vi "Create or Load Experiment Dialog.vi"(8 "error in (no error)":errorcluster, 11 "User Preferences File.lvclass":refnum<class "User Preferences File.lvclass">) -> (0 "error out":errorcluster, 1 "Cancelled?":bool, 2 "Experimental File Cluster":T1, 3 "Experiment File Path":path, 4 "Experiment File Extension":string, 5 "Experiment Name":string)   [LabVIEW 2020, in "RxnRover.lvlib" / "Experiment Manager.lvlib"]
uses:
  Experiment Manager.lvlib
  Experiment File/Experiment File Cluster.ctl
  Plugin Servers/Controller/Minimal Controller Cluster.ctl
  Plugin Servers/Parameter to Hardware Map/Minimal Map.ctl
  Plugin Servers/Parameter to Hardware Map/Minimal Pair Cluster.ctl
  UI Data.ctl
  Sub VIs/Message Queue/Enqueue Message (Single).vi
  <vilib>/Utility/error.llb/Error Cluster From Error Code.vi
  <vilib>/ErrorRing/Error Ring.xnode
  User Preferences/User Preferences File.lvclass
  Sub VIs/Message Queue/test Message Queue.lvlib
  User Event - Stop/User Event - Stop.lvlib
  Plugin Servers/Controller/Generic Plugin.lvclass
  Experiment File/Experiment File.lvlib
  Plugin Servers/Parameter to Hardware Map/Parameter to Hardware Map.lvclass
panel:
  in  "Continue Without Experiment Btn":bool
  in  "Load Experiment Btn":bool
  in  "New Experiment Btn":bool
  in  "Clear Recent Experiments Button":bool
  in  "Recent Experiments Listbox":i32(listbox)
  # "Create or Load Experiment"
  # "Experiment Options"
  # "Recent Experiments"
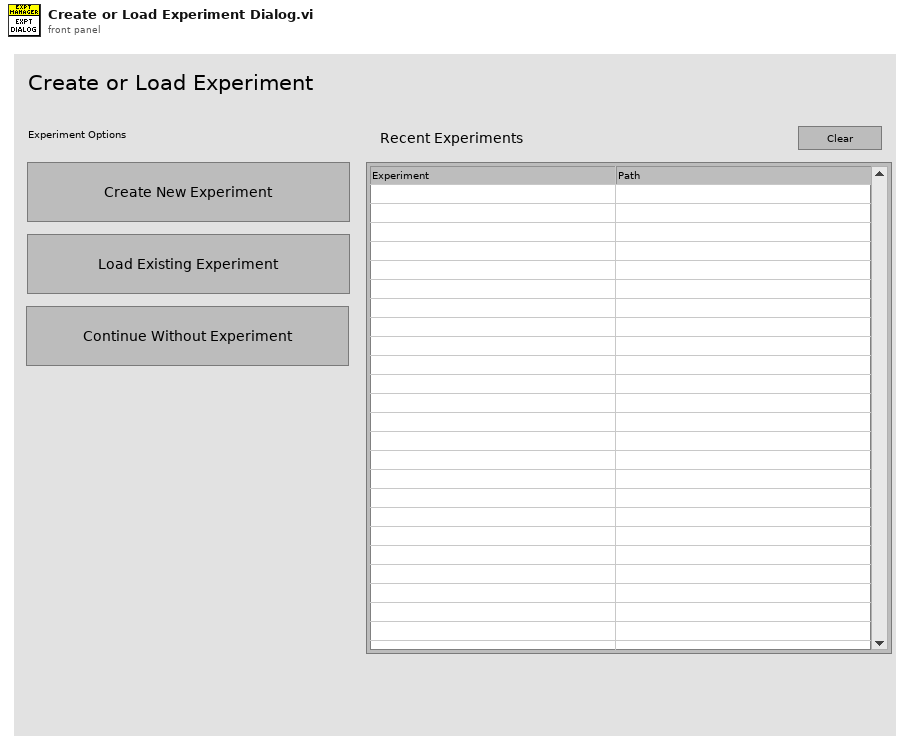
[diagram p1: front panel]
types:
  T1 = typedef "RxnRover.lvlib/Experiment File.lvlib/Experiment File Cluster.ctl" = cluster{"Hardware List":T2[], "Optimizer List":T2[], "Analyzer List":T2[], "Parameter to Hardware Map":T3}
  T2 = typedef "RxnRover.lvlib/Generic Plugin.lvclass/Minimal Controller Cluster.ctl" = cluster{"Name":string, "Controller Type":string, "Control Panel Path":string, "Resource":string}
  T3 = typedef "RxnRover.lvlib/Parameter to Hardware Map.lvclass/Minimal Map.ctl" = T4[]
  T4 = typedef "RxnRover.lvlib/Parameter to Hardware Map.lvclass/Minimal Pair Cluster.ctl" = cluster{"key":string, "values":T2[]}
  T5 = typedef "RxnRover.lvlib/Experiment Manager.lvlib/UI Data.ctl" = cluster{"New Project Btn":refnum<vi>, "Load Project Btn":refnum<vi>, "Cancelled?":bool, "Experiment File Path":path, "Experiment File":T1, "Experiment Directory":path, "Experiment Name":string, "Experiment File Extension":string, "User Preferences File":refnum<class "User Preferences File.lvclass">, "Recent Experiments Listbox":refnum<vi>}
  T6 = enum32{"Invalid", "Standard", "Closed", "Hidden", "Minimized", "Maximized"}
  T7 = typedef "RxnRover.lvlib/User Preferences File.lvclass/User Preferences Cluster.ctl" = cluster{"Max Recent Experiments":dbl, "Recent Experiments":string[], "Log Level":string}
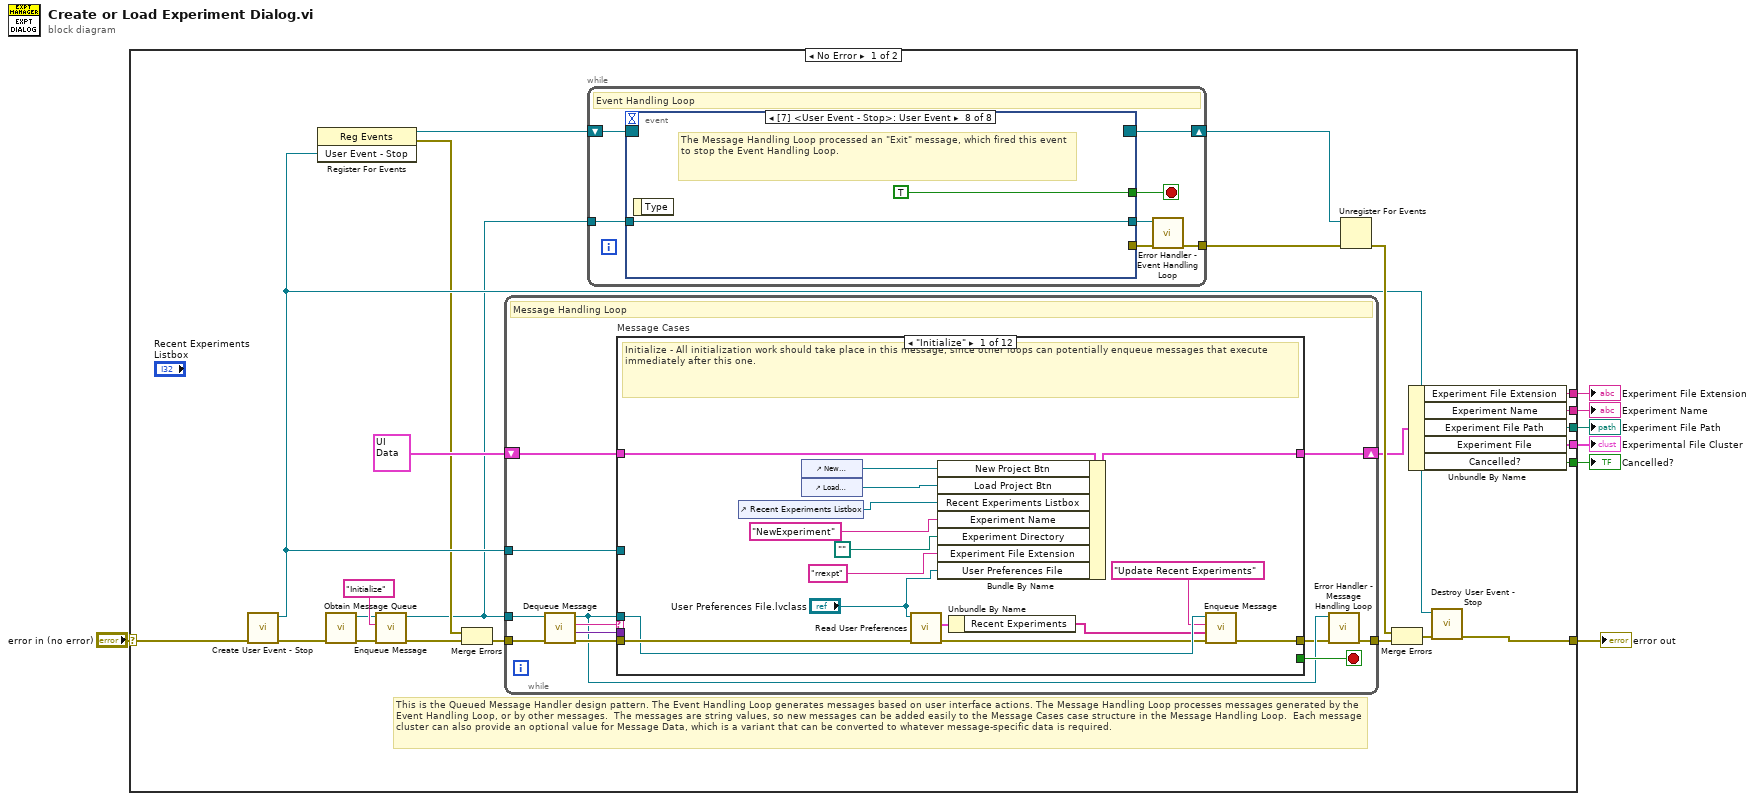
[diagram p0: block diagram]
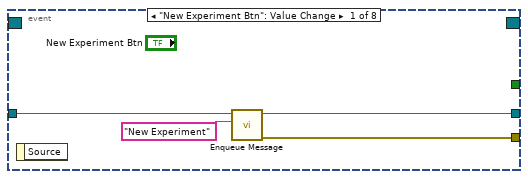
[diagram p2: hidden frame]
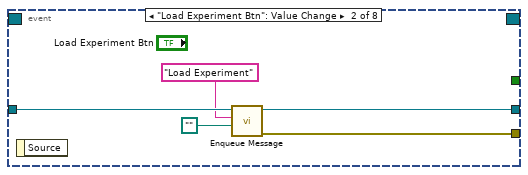
[diagram p3: hidden frame]
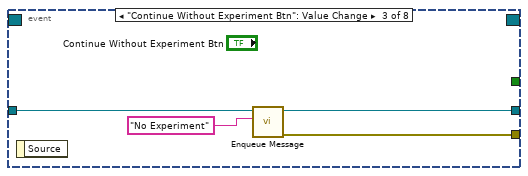
[diagram p4: hidden frame]
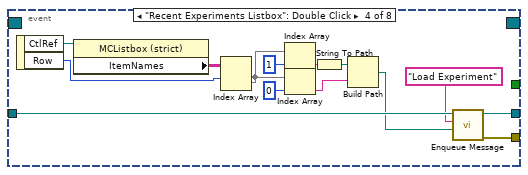
[diagram p5: hidden frame]
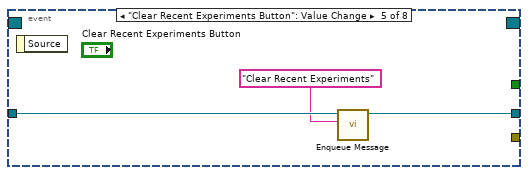
[diagram p6: hidden frame]
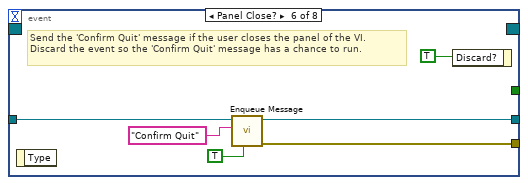
[diagram p7: hidden frame]
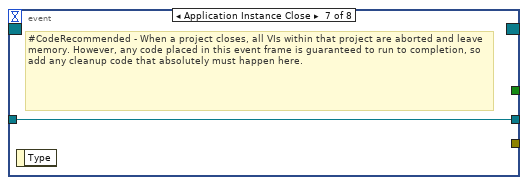
[diagram p8: hidden frame]
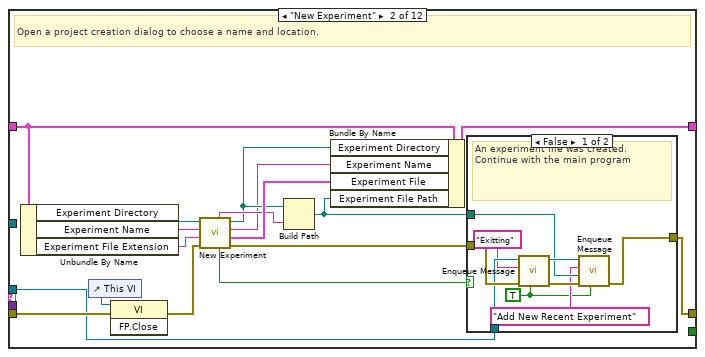
[diagram p9: hidden frame]
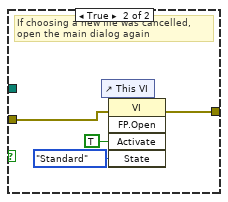
[diagram p10: hidden frame]
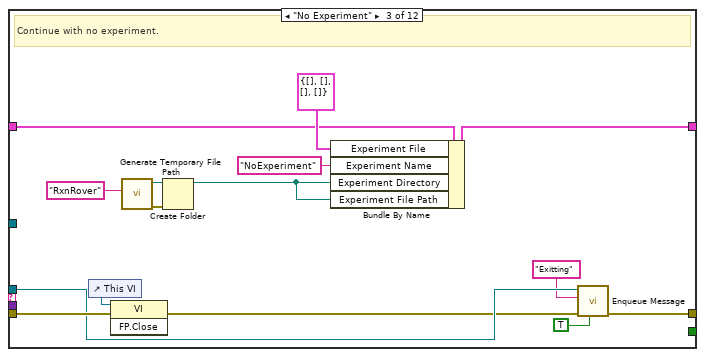
[diagram p11: hidden frame]
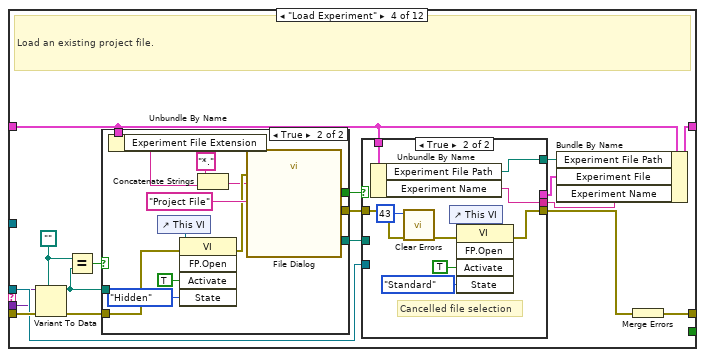
[diagram p12: hidden frame]
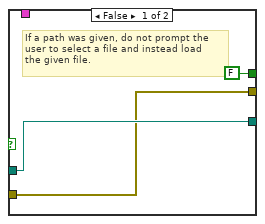
[diagram p13: hidden frame]
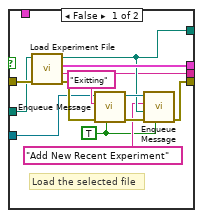
[diagram p14: hidden frame]
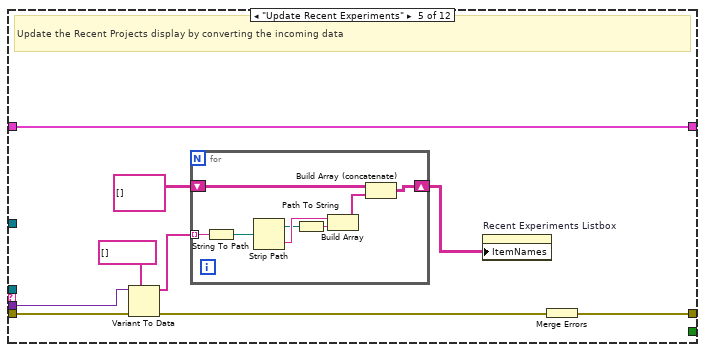
[diagram p15: hidden frame]
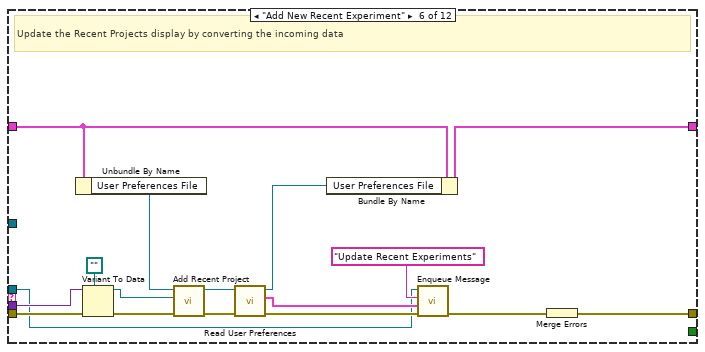
[diagram p16: hidden frame]
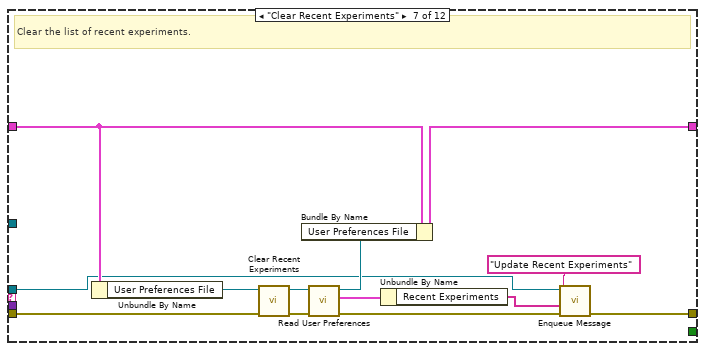
[diagram p17: hidden frame]
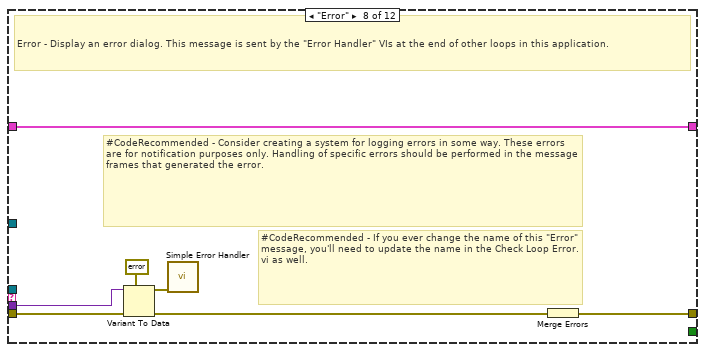
[diagram p18: hidden frame]
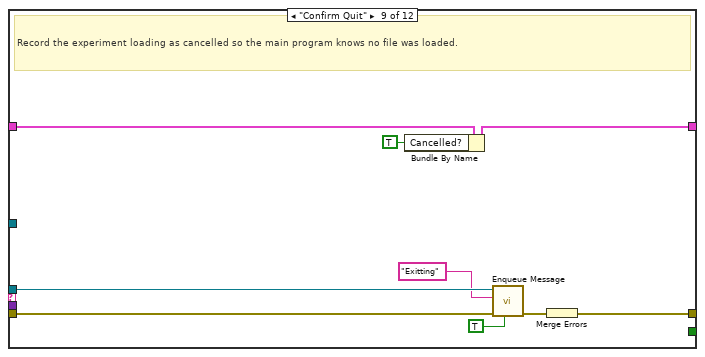
[diagram p19: hidden frame]
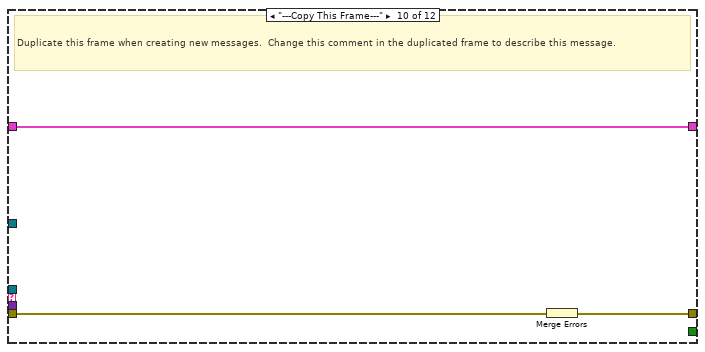
[diagram p20: hidden frame]
diagram:
  n1 = case shown="No Error" "error in (no error)" {
    selector: "error in (no error)" -> [w11 w301]
    tunnel: [w15 w301] -> w1
    tunnel: [w13 T1 {"Hardware List"=[], "Optimizer List"=[], "Analyzer List"=[], "Parameter to Hardware Map"=[]} ("File")] -> w7
    tunnel: [w12 TRUE ("Cancelled?")] -> w6
    tunnel: [w10 path ""] -> w4
    tunnel: [w9 w297] -> w3
    tunnel: [w8 w297] -> w2
    frame No Error {
      # "This is the Queued Message Handler design pattern. The Event Handling Loop generates messages based on user interface actions. The Message Handling Loop processes messages generated by the Event Handling Loop, or by other messages.  The messages are string values, so new messages can be added easily to the Message Cases case structure in the Message Handling Loop.  Each message cluster can also provide an optional value for Message Data, which is a variant that can be converted to whatever message-specific data is required."
      n2 = call "Create User Event - Stop.vi"("error in (no error)"=w11) -> ("error out"=w21:errorcluster, "User Event - Stop"=w24:refnum<user-event>)  [unwired: 9 in]
      n3 = register-events(w24) -> (reference out=w25:refnum<event-registration>, error out=w22:errorcluster)  [unwired: 2 in]
      n4 = call "Obtain Message Queue.vi"("error in (no error)"=w21) -> ("error out"=w20:errorcluster, "Message Queue"=w17:refnum<queue>)  [unwired: 9 in]
      n5 = call-poly "Enqueue Message.vi"("error in (no error)"=w20, "Message"="Initialize", "Message Queue"=w17) -> ("error out"=w19:errorcluster, "dup Message Queue"=w16:refnum<queue>)  [unwired: 7 in]
      n6 = Merge Errors(w22, w19) -> (w23:errorcluster)
      n7 = while {
        tunnel: w16 -> [w81]
        shift-right: [w88] -> w14
        shift-left: T5 {"New Project Btn"=refnum, "Load Project Btn"=refnum, "Cancelled?"=FALSE, "Experiment File Path"=path "", "Experiment File"={"Hardware List"=[], "Optimizer List"=[], "Analyzer List"=[], "Parameter to Hardware Map"=[]}, "Experiment Directory"=path "", "Experiment Name"="", "Experiment File Extension"="", "User Preferences File"=refnum, "Recent Experiments Listbox"=refnum} ("Data Cluster") -> [w89]
        tunnel: w24 -> [w86]
        tunnel: w23 -> [w85]
        tunnel: [w79] -> w31
        stop <- w87 stop-if-true
        # "Message Handling Loop"
        n8 = call "Dequeue Message.vi"("error in (no error)"=w85, "Message Queue"=w81) -> ("error out"=w84:errorcluster, "Message Data"=w82:variant, "Message"=w83:string, "dup Message Queue"=w80:refnum<queue>)  [unwired: 6 in]
        n9 = case "Message Cases" shown="\"Initialize\"" w83 {
          selector: w83 -> [_ _ _ _ _ _ _ _ _ _ _ w287]
          tunnel: w80 -> [w99 w116 w148 w158 _ w226 w244 _ w266 _ w286 _]
          tunnel: w84 -> [w104 w120 w149 w162 w214 w240 w254 w261 w270 w273 w280 _]
          tunnel: [w105 w117 w145 w168 w215 w241 w245 w255 w268 w271 w283 w288] -> w78
          tunnel: w89 -> [w103 w115 w139 w159 w216 w237 w253 w260 w269 w272 w276 w289]
          tunnel: [w102 w122 w151 w163 w216 w232 w251 w260 w263 w272 w276 w289] -> w88
          tunnel: [_ _ _ _ _ _ _ _ _ _ TRUE _] -> w87
          tunnel: w82 -> [_ _ _ w156 w213 w239 _ w259 _ _ w277 _]
          tunnel: w86 -> [_ _ _ _ _ _ _ _ _ _ w282 _]
          frame "Initialize" {
            # "Initialize - All initialization work should take place in this message, since other loops can potentially enqueue messages that execute immediately after this one."
            n10 = control-ref of="Recent Experiments Listbox"() -> (w91:refnum<vi>)
            n11 = control-ref of="New Experiment Btn"() -> (w101:refnum<vi>)
            n12 = control-ref of="Load Experiment Btn"() -> (w100:refnum<vi>)
            n13 = call-dynamic "Read User Preferences.vi"("error in (no error)"=w104, "User Preferences File in"="User Preferences File.lvclass") -> ("error out"=w94:errorcluster, "User Preferences"=w93:T7)  [unwired: 7 in, 1 out]
            n14 = Bundle By Name(cluster=w103, "New Project Btn"=w101, "Load Project Btn"=w100, "Recent Experiments Listbox"=w91, "Experiment Name"="NewExperiment", "Experiment Directory"=path "", "Experiment File Extension"="rrexpt", "User Preferences File"="User Preferences File.lvclass") -> (w102:T5)
            n15 = Unbundle By Name(w93) -> ("Recent Experiments"=w92:string[])
            n16 = call-poly "Enqueue Message.vi"("error in (no error)"=w94, "Message Data"=w92, "Message"="Update Recent Experiments", "Message Queue"=w99) -> ("error out"=w105:errorcluster)  [unwired: 6 in, 1 out]
          }
          frame "New Experiment" {
            # "Open a project creation dialog to choose a name and location."
            n17 = Unbundle By Name(w115) -> ("Experiment Directory"=w113:path, "Experiment Name"=w107:string, "Experiment File Extension"=w109:string)
            n18 = control-ref of="This VI"() -> (w121:refnum<vi>)
            n19 = invoke class="VI" method="FP.Close"(reference=w121, error in=w120) -> (error out=w119:errorcluster)  [unwired: 1 in, 2 out]
            n20 = call "New Experiment.vi"("error in (no error)"=w119, "Experiment File Extension"=w109, "Experiment Name in"=w107, "Experiment Location in"=w113) -> ("error out"=w118:errorcluster, "Experiment File Cluster"=w112:T1, "Experiment Name out"=w106:string, "Experiment Location out"=w110:path, "cancelled"=w114:bool, "Experiment filename out"=w111:string)  [unwired: 2 in]
            n21 = Build Path(base path=w110, name or relative path=w111) -> (appended path=w108:path)
            n22 = Bundle By Name(cluster=w115, "Experiment Directory"=w110, "Experiment Name"=w106, "Experiment File"=w112, "Experiment File Path"=w108) -> (w122:T5)
            n23 = case shown="False" w114 {
              tunnel: w118 -> [w131 w135]
              tunnel: [w127 w134] -> w117
              tunnel: w116 -> [w130 _]
              tunnel: w108 -> [w125 _]
              frame False {
                w123 = TRUE ("Priority Message? (F)")
                # "An experiment file was created. Continue with the main program"
                n24 = call-poly "Enqueue Message.vi"("Priority Message? (F)"=w123, "error in (no error)"=w131, "Message"="Exitting", "Message Queue"=w130) -> ("error out"=w128:errorcluster, "dup Message Queue"=w126:refnum<queue>)  [unwired: 6 in]
                n25 = call-poly "Enqueue Message.vi"("Priority Message? (F)"=w123, "error in (no error)"=w128, "Message Data"=w125, "Message"="Add New Recent Experiment", "Message Queue"=w126) -> ("error out"=w127:errorcluster)  [unwired: 5 in, 1 out]
              }
              frame True {
                # "If choosing a new file was cancelled, open the main dialog again"
                n26 = control-ref of="This VI"() -> (w136:refnum<vi>)
                n27 = invoke class="VI" method="FP.Open"(reference=w136, error in=w135, "Activate"=TRUE ("Activate?"), "State"=T6."Standard") -> (error out=w134:errorcluster)  [unwired: 1 in, 4 out]
              }
            }
          }
          frame "No Experiment" {
            # "Continue with no experiment."
            n28 = control-ref of="This VI"() -> (w150:refnum<vi>)
            n29 = invoke class="VI" method="FP.Close"(reference=w150, error in=w149) -> (error out=w141:errorcluster)  [unwired: 1 in, 2 out]
            n30 = call <vilib>:"Generate Temporary File Path.vi"("Temporary File Extension (tmp)"="RxnRover") -> ("error out"=w143:errorcluster, "Unique Temporary File Path"=w144:path)  [unwired: 9 in]
            n31 = Create Folder(path (use dialog)=w144, error in=w143) -> (created path=w137:path)  [unwired: 1 in, 2 out]
            n32 = Bundle By Name(cluster=w139, "Experiment File"=T1 {"Hardware List"=[], "Optimizer List"=[], "Analyzer List"=[], "Parameter to Hardware Map"=[]} ("Experiment File Cluster"), "Experiment Name"="NoExperiment", "Experiment Directory"=w137, "Experiment File Path"=w137) -> (w151:T5)
            n33 = call-poly "Enqueue Message.vi"("Priority Message? (F)"=TRUE, "error in (no error)"=w141, "Message"="Exitting", "Message Queue"=w148) -> ("error out"=w145:errorcluster)  [unwired: 6 in, 1 out]
          }
          frame "Load Experiment" {
            w154 = path ""
            # "Load an existing project file."
            n34 = Variant To Data(error in=w162, type=w154, Variant=w156) -> (data=w153:path, error out=w157:errorcluster)
            n35 = Equal?(x=w154, y=w153) -> (x = y?=w155:bool)
            n36 = case shown="True" w155 {
              tunnel: [FALSE ("cancelled") w183] -> w167
              tunnel: [w169 w182] -> w166
              tunnel: [w171 w181] -> w164
              tunnel: w157 -> [w169 w180]
              tunnel: w159 -> [_ w175]
              tunnel: w153 -> [w171 _]
              frame False {
                # "If a path was given, do not prompt the\nuser to select a file and instead load\nthe given file."
              }
              frame True {
                n37 = Unbundle By Name(w175) -> ("Experiment File Extension"=w173:string)
                n38 = control-ref of="This VI"() -> (w178:refnum<vi>)
                n39 = invoke class="VI" method="FP.Open"(reference=w178, error in=w180, "Activate"=TRUE ("Activate?"), "State"=T6."Hidden") -> (error out=w179:errorcluster)  [unwired: 1 in, 4 out]
                n40 = Concatenate Strings("*." ("pattern (all files)"), w173) -> (w174:string)
                n41 = call "File Dialog"("button label"="Project File", "error in"=w179, "pattern (all files)"=w174) -> ("selected path"=w181:path, "cancelled"=w183:bool, "error out"=w182:errorcluster)  [unwired: 9 in, 1 out]
              }
            }
            n42 = case shown="True" w167 {
              tunnel: w166 -> [w197 w202]
              tunnel: [w190 w204] -> w165
              tunnel: w164 -> [w196 _]
              tunnel: [w192 _] -> w161
              tunnel: w158 -> [w193 _]
              tunnel: [w188 w199] -> w160
              tunnel: w159 -> [_ w200]
              tunnel: [w185 w198] -> w152
              frame False {
                w186 = TRUE ("Priority Message? (F)")
                # "Load the selected file"
                n43 = call "Load Experiment File.vi"("error in (no error)"=w197, "Experiment File Path"=w196) -> ("error out"=w194:errorcluster, "Experiment Name"=w185:string, "Experiment File out"=w192:T1, "Experiment File Path out (duplicate)"=w188:path)  [unwired: 6 in]
                n44 = call-poly "Enqueue Message.vi"("Priority Message? (F)"=w186, "error in (no error)"=w194, "Message"="Exitting", "Message Queue"=w193) -> ("error out"=w191:errorcluster, "dup Message Queue"=w189:refnum<queue>)  [unwired: 6 in]
                n45 = call-poly "Enqueue Message.vi"("Priority Message? (F)"=w186, "error in (no error)"=w191, "Message Data"=w188, "Message"="Add New Recent Experiment", "Message Queue"=w189) -> ("error out"=w190:errorcluster)  [unwired: 5 in, 1 out]
              }
              frame True {
                # "Cancelled file selection"
                n46 = Unbundle By Name(w200) -> ("Experiment File Path"=w199:path, "Experiment Name"=w198:string)
                n47 = call <vilib>:"Clear Errors.vi"("error in (no error)"=w202, "specific error code to clear (0: all)"=43) -> ("error out"=w201:errorcluster)  [unwired: 4 in, 1 out]
                n48 = control-ref of="This VI"() -> (w207:refnum<vi>)
                n49 = invoke class="VI" method="FP.Open"(reference=w207, error in=w201, "Activate"=TRUE ("Activate?"), "State"=T6."Standard") -> (error out=w204:errorcluster)  [unwired: 1 in, 4 out]
              }
            }
            n50 = Bundle By Name(cluster=w159, "Experiment File Path"=w160, "Experiment File"=w161, "Experiment Name"=w152) -> (w163:T5)
            n51 = Merge Errors(w165) -> (w168:errorcluster)
          }
          frame "Update Recent Experiments" {
            # "Update the Recent Projects display by converting the incoming data"
            n52 = Variant To Data(error in=w214, type=string[] [], Variant=w213) -> (data=w210:string[], error out=w212:errorcluster)
            n53 = for {
              tunnel: w210 -> [w224] mode=indexing
              shift-right: [w222] -> w208
              shift-left: string[][] [] -> [w223]
              n54 = String To Path(string=w224) -> (path=w217:path)
              n55 = Strip Path(path=w217) -> (stripped path=w220:path, name=w221:string)
              n56 = Path To String(path=w220) -> (string=w218:string)
              n57 = Build Array(w221, w218) -> (w219:string[])
              n58 = Build Array (concatenate)(w223, w219) -> (w222:string[][])
            }
            n59 = property on="Recent Experiments Listbox" class="MCListbox (strict)"("ItemNames"=w208) -> ()  [unwired: 2 in, 2 out]
            n60 = Merge Errors(w212) -> (w215:errorcluster)
          }
          frame "Add New Recent Experiment" {
            # "Update the Recent Projects display by converting the incoming data"
            n61 = Unbundle By Name(w237) -> ("User Preferences File"=w235:refnum<class "User Preferences File.lvclass">)
            n62 = Variant To Data(error in=w240, type=path "", Variant=w239) -> (data=w225:path, error out=w236:errorcluster)
            n63 = call "Add Recent Project.vi"("error in (no error)"=w236, "New Recent Experiment path"=w225, "User Preferences File in"=w235) -> ("error out"=w234:errorcluster, "User Preferences File out"=w233:refnum<class "User Preferences File.lvclass">)  [unwired: 7 in]
            n64 = call-dynamic "Read User Preferences.vi"("error in (no error)"=w234, "User Preferences File in"=w233) -> ("error out"=w230:errorcluster, "User Preferences"=w228:T7, "User Preferences File out"=w231:refnum<class "User Preferences File.lvclass">)  [unwired: 7 in]
            n65 = Bundle By Name(cluster=w237, "User Preferences File"=w231) -> (w232:T5)
            n66 = call-poly "Enqueue Message.vi"("error in (no error)"=w230, "Message Data"=w228, "Message"="Update Recent Experiments", "Message Queue"=w226) -> ("error out"=w229:errorcluster)  [unwired: 6 in, 1 out]
            n67 = Merge Errors(w229) -> (w241:errorcluster)
          }
          frame "Clear Recent Experiments" {
            # "Clear the list of recent experiments."
            n68 = Unbundle By Name(w253) -> ("User Preferences File"=w252:refnum<class "User Preferences File.lvclass">)
            n69 = call "Clear Recent Experiments.vi"("error in (no error)"=w254, "User Preferences File in"=w252) -> ("error out"=w248:errorcluster, "User Preferences File out"=w250:refnum<class "User Preferences File.lvclass">)  [unwired: 8 in]
            n70 = call-dynamic "Read User Preferences.vi"("error in (no error)"=w248, "User Preferences File in"=w250) -> ("error out"=w246:errorcluster, "User Preferences"=w247:T7, "User Preferences File out"=w249:refnum<class "User Preferences File.lvclass">)  [unwired: 7 in]
            n71 = Bundle By Name(cluster=w253, "User Preferences File"=w249) -> (w251:T5)
            n72 = Unbundle By Name(w247) -> ("Recent Experiments"=w243:string[])
            n73 = call-poly "Enqueue Message.vi"("error in (no error)"=w246, "Message Data"=w243, "Message"="Update Recent Experiments", "Message Queue"=w244) -> ("error out"=w245:errorcluster)  [unwired: 6 in, 1 out]
          }
          frame "Error" {
            # "#CodeRecommended - If you ever change the name of this \"Error\" message, you'll need to update the name in the Check Loop Error.vi as well."
            # "#CodeRecommended - Consider creating a system for logging errors in some way. These errors are for notification purposes only. Handling of specific errors should be performed in the message frames that generated the error."
            # "Error - Display an error dialog. This message is sent by the \"Error Handler\" VIs at the end of other loops in this application."
            n74 = Variant To Data(error in=w261, type=errorcluster {"status"=FALSE, "code"=0, "source"=""} ("error constant"), Variant=w259) -> (data=w257:errorcluster, error out=w256:errorcluster)
            n75 = call <vilib>:"Simple Error Handler.vi"("error in (no error)"=w257) -> ()  [unwired: 4 in, 5 out]
            n76 = Merge Errors(w256) -> (w255:errorcluster)
          }
          frame "Confirm Quit" {
            # "Record the experiment loading as cancelled so the main program knows no file was loaded."
            n77 = Bundle By Name(cluster=w269, "Cancelled?"=TRUE) -> (w263:T5)
            n78 = call-poly "Enqueue Message.vi"("Priority Message? (F)"=TRUE, "error in (no error)"=w270, "Message"="Exitting", "Message Queue"=w266) -> ("error out"=w267:errorcluster)  [unwired: 6 in, 1 out]
            n79 = Merge Errors(w267) -> (w268:errorcluster)
          }
          frame "---Copy This Frame---" {
            # "Duplicate this frame when creating new messages.  Change this comment in the duplicated frame to describe this message."
            n80 = Merge Errors(w273) -> (w271:errorcluster)
          }
          frame "Exitting" {
            # "Stop the VI"
            # "Release the message queue reference"
            # "Exit - Exit the application."
            n81 = Unbundle By Name(w276) -> ("User Preferences File"=w275:refnum<class "User Preferences File.lvclass">)
            n82 = Variant To Data(type=errorcluster {"status"=FALSE, "code"=0, "source"=""} ("error constant"), Variant=w277) -> (data=w278:errorcluster)  [unwired: 1 in, 1 out]
            n83 = call <vilib>:"Simple Error Handler.vi"("error in (no error)"=w278) -> ()  [unwired: 4 in, 5 out]
            n84 = call "Fire User Event - Stop.vi"("User Event - Stop"=w282) -> ("error out"=w281:errorcluster)  [unwired: 10 in]
            n85 = call "Save.vi"("User Preferences File in"=w275) -> ("error out"=w274:errorcluster)  [unwired: 9 in, 1 out]
            n86 = Release Queue(queue=w286, error in (no error)=w280) -> (error out=w284:errorcluster)  [unwired: 1 in, 2 out]
            n87 = Merge Errors(w274, w281, w284) -> (w283:errorcluster)
          }
          frame Default {
            # "'Default' case only runs if there is a message that isn't defined in any of the other cases.  Output a programming error."
            n88 = xnode "Error Ring"("parameter 0"=w287) -> ("error out"=w288:errorcluster)
          }
        }
        n89 = call "Error Handler - Message Handling Loop.vi"("error in (no error)"=w78, "Message Queue"=w80) -> ("dup error in"=w79:errorcluster)  [unwired: 8 in, 1 out]
      }
      n90 = while {
        tunnel: w16 -> [w38]
        shift-right: [w36] -> w28
        shift-left: w25 -> [w37]
        tunnel: [w32] -> w26
        stop <- w34 stop-if-true
        # "Event Handling Loop"
        n91 = event shown="[7] <User Event - Stop>: User Event" {
          selector: w37 -> [_ _ _ _ _ _ _ _]
          dyn-events: [_ _ _ _ _ _ _ _] -> w36
          timeout: _ -> [_ _ _ _ _ _ _ _]
          tunnel: [_ _ _ _ _ _ _ TRUE ("Discard?")] -> w34
          tunnel: w38 -> [w42 w47 w50 w65 w68 w73 w75 w77]
          tunnel: [w39 w44 w48 w63 _ w72 _ _] -> w35
          tunnel: [w41 w46 w49 w64 w67 w71 w75 w77] -> w33
          event "New Experiment Btn": Value Change {
            n92 = event-data() -> ()  [unwired: 1 in, 1 out]
            n93 = call-poly "Enqueue Message.vi"("Message"="New Experiment", "Message Queue"=w42) -> ("error out"=w39:errorcluster, "dup Message Queue"=w41:refnum<queue>)  [unwired: 8 in]
          }
          event "Load Experiment Btn": Value Change {
            n94 = event-data() -> ()  [unwired: 1 in, 1 out]
            n95 = call-poly "Enqueue Message.vi"("Message Data"=path "", "Message"="Load Experiment", "Message Queue"=w47) -> ("error out"=w44:errorcluster, "dup Message Queue"=w46:refnum<queue>)  [unwired: 7 in]
          }
          event "Continue Without Experiment Btn": Value Change {
            n96 = event-data() -> ()  [unwired: 1 in, 1 out]
            n97 = call-poly "Enqueue Message.vi"("Message"="No Experiment", "Message Queue"=w50) -> ("error out"=w48:errorcluster, "dup Message Queue"=w49:refnum<queue>)  [unwired: 8 in]
          }
          event "Recent Experiments Listbox": Double Click {
            n98 = event-data() -> ("CtlRef"=w61:refnum<vi>, "Row"=w59:i32)  [unwired: 1 in]
            n99 = property class="MCListbox (strict)"(reference=w61) -> ("ItemNames"=w60:string[][])  [unwired: 1 in, 2 out]
            n100 = Index Array(array=w60, index (row)=w59) -> (element=w58:string[])  [unwired: 1 in]
            n101 = Index Array(array=w58, index=1) -> (element=w55:string)
            n102 = Index Array(array=w58, index=0) -> (element=w54:string)
            n103 = String To Path(string=w55) -> (path=w53:path)
            n104 = Build Path(base path=w53, name or relative path=w54) -> (appended path=w52:path)
            n105 = call-poly "Enqueue Message.vi"("Message Data"=w52, "Message"="Load Experiment", "Message Queue"=w65) -> ("error out"=w63:errorcluster, "dup Message Queue"=w64:refnum<queue>)  [unwired: 7 in]
          }
          event "Clear Recent Experiments Button": Value Change {
            n106 = event-data() -> ()  [unwired: 1 in, 1 out]
            n107 = call-poly "Enqueue Message.vi"("Message"="Clear Recent Experiments", "Message Queue"=w68) -> ("dup Message Queue"=w67:refnum<queue>)  [unwired: 8 in, 1 out]
          }
          event Panel Close? {
            # "Send the 'Confirm Quit' message if the user closes the panel of the VI. Discard the event so the 'Confirm Quit' message has a chance to run."
            n108 = event-data() -> ()  [unwired: 1 in, 1 out]
            n109 = call-poly "Enqueue Message.vi"("Priority Message? (F)"=TRUE, "Message"="Confirm Quit", "Message Queue"=w73) -> ("error out"=w72:errorcluster, "dup Message Queue"=w71:refnum<queue>)  [unwired: 7 in]
            n110 = event-data("Discard?"=TRUE) -> ()  [unwired: 1 in, 1 out]
          }
          event Application Instance Close {
            # "#CodeRecommended - When a project closes, all VIs within that project are aborted and leave memory. However, any code placed in this event frame is guaranteed to run to completion, so add any cleanup code that absolutely must happen here."
            n111 = event-data() -> ()  [unwired: 1 in, 1 out]
          }
          event User Event {
            # "The Message Handling Loop processed an \"Exit\" message, which fired this event to stop the Event Handling Loop."
            n112 = event-data() -> ()  [unwired: 1 in, 1 out]
          }
        }
        n113 = call "Error Handler - Event Handling Loop.vi"("error in (no error)"=w35, "Message Queue"=w33) -> ("dup error in"=w32:errorcluster)  [unwired: 8 in, 1 out]
      }
      n114 = Unregister For Events(event registration refnum=w28, error in=w26) -> (error out=w29:errorcluster)
      n115 = Merge Errors(w29, w31) -> (w30:errorcluster)
      n116 = Unbundle By Name(w14) -> ("Experiment File Extension"=w8:string, "Experiment Name"=w9:string, "Experiment File Path"=w10:path, "Experiment File"=w13:T1, "Cancelled?"=w12:bool)
      n117 = call "Destroy User Event - Stop.vi"("error in (no error)"=w30, "User Event - Stop"=w24) -> ("error out"=w15:errorcluster)  [unwired: 9 in]
    }
    frame Error {
      w297 = ""
    }
  }
  "error out" <- w1
  "Experimental File Cluster" <- w7
  "Cancelled?" <- w6
  "Experiment File Path" <- w4
  "Experiment Name" <- w3
  "Experiment File Extension" <- w2
